vi "Read Data_HoldingRegistors.vi"(8 "error in (no error)":errorcluster, 11 "Device in":refnum<class "MB_TCP_Device.lvclass">) -> (0 "error out":errorcluster, 2 "AI Data":dbl[](array[numeric]), 3 "Device out":refnum<class "MB_TCP_Device.lvclass">)   [LabVIEW 2023, in "MB_TCP_Device.lvclass"]
uses:
  MB_TCP_Device.lvclass
  MB_TCP_Device.lvclass/MB_TCP_Device.ctl
  <vilib>/NI Modbus.llb/MB Ethernet Master Query Read Holding Registers (poly).vi
  <vilib>/Utility/error.llb/Error Cluster From Error Code.vi
  <vilib>/ErrorRing/Error Ring.xnode
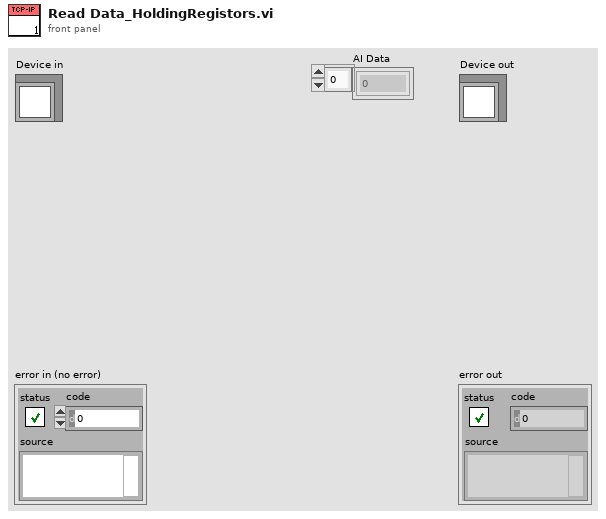
[diagram p1: front panel]
types:
  T1 = typedef "DAQ Device_IO ChannelsData.ctl" = cluster{"#DigitalInputs":u16, "StartAddress_DI":u16, "#DigitalOutputs":u16, "StartAddress_DO":u16, "#AnalogInputs":u16, "StartAddress_AI":u16, "#AnalogOutputs":u16, "StartAddress_AO":u16, "Coil_ReadData":bool[], "Coil_WriteData":bool[], "AI_Data":u16[], "AO_Data":u16[]}
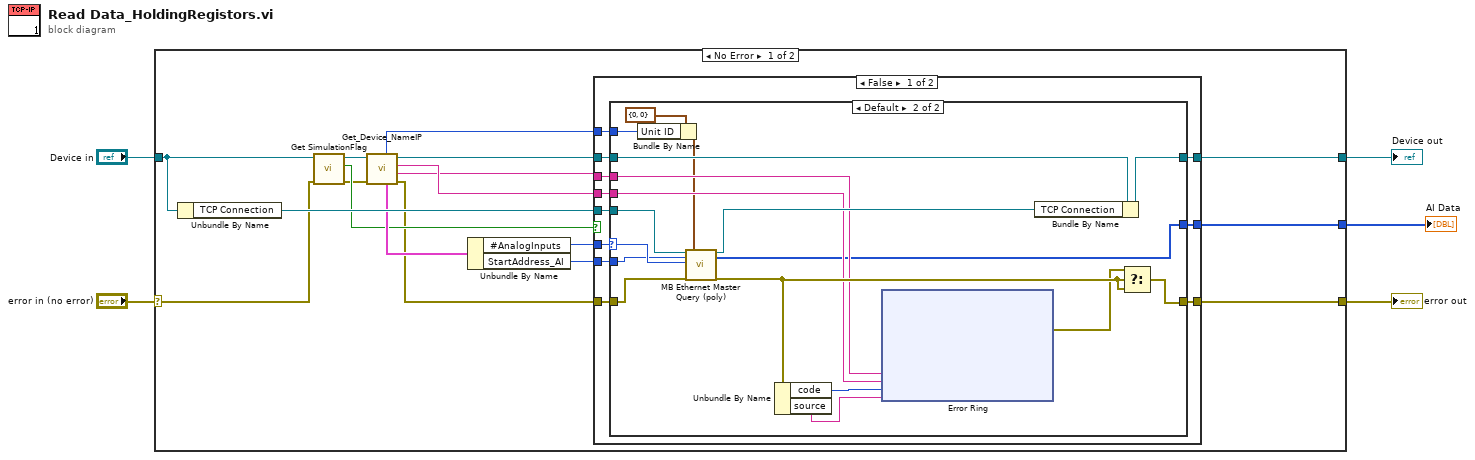
[diagram p0: block diagram]
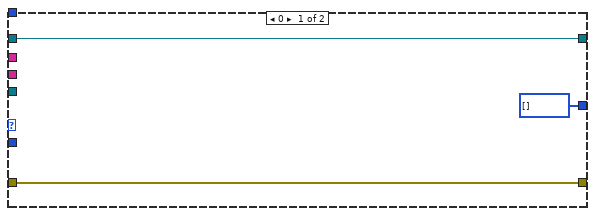
[diagram p2: hidden frame]
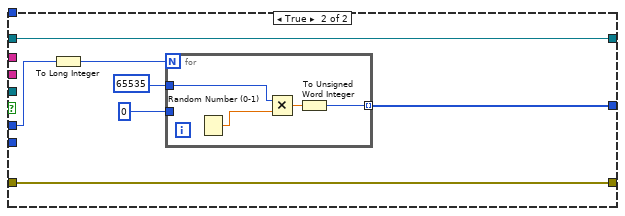
[diagram p3: hidden frame]
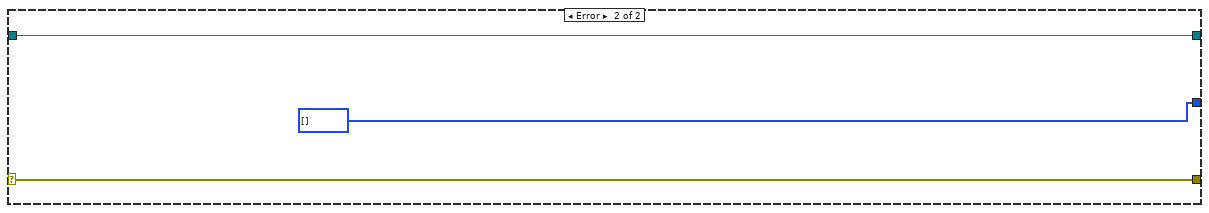
[diagram p4: hidden frame]
diagram:
  n1 = case shown="No Error" "error in (no error)" {
    selector: "error in (no error)" -> [w8 w78]
    tunnel: [w21 w78] -> w4
    tunnel: [w22 w77] -> w2
    tunnel: "Device in" -> [w14 w77]
    tunnel: [w6 u16[] [] ("register values")] -> w1
    frame No Error {
      n2 = Unbundle By Name(w14) -> ("TCP Connection"=w20:refnum<k5>)
      n3 = call-dynamic "Get SimulationFlag.vi"("error in (no error)"=w8, "Device in"=w14) -> ("error out"=w9:errorcluster, "Simulation?"=w12:bool, "Device out"=w15:refnum<class "MB_TCP_Device.lvclass">)  [unwired: 7 in]
      n4 = call-dynamic "Get_Device_NameIP.vi"("error in (no error)"=w9, "Device in"=w15) -> ("error out"=w7:errorcluster, "Device Name"=w17:string, "Device Address"=w18:string, "Device out"=w13:refnum<class "MB_TCP_Device.lvclass">, "IO Channels"=w19:T1, "Unit ID"=w16:u8)  [unwired: 4 in]
      n5 = Unbundle By Name(w19) -> ("#AnalogInputs"=w11:u16, "StartAddress_AI"=w10:u16)
      n6 = case shown="False" w12 {
        tunnel: [w33 w66] -> w22
        tunnel: w7 -> [w32 w71]
        tunnel: w11 -> [w25 w68]
        tunnel: w10 -> [w31 _]
        tunnel: [w30 w71] -> w21
        tunnel: w20 -> [w29 _]
        tunnel: w18 -> [w26 _]
        tunnel: w13 -> [w28 w66]
        tunnel: w17 -> [w27 _]
        tunnel: w16 -> [w24 _]
        tunnel: [w23 w65] -> w6
        frame False {
          n7 = case shown="Default" w25 {
            selector: w25 -> [_ w42]
            tunnel: [w36 w54] -> w33
            tunnel: w32 -> [w35 w52]
            tunnel: w31 -> [_ w41]
            tunnel: [w35 w50] -> w30
            tunnel: w29 -> [_ w49]
            tunnel: w28 -> [w36 w48]
            tunnel: w27 -> [_ w47]
            tunnel: w26 -> [_ w46]
            tunnel: w24 -> [_ w38]
            tunnel: [u16[] [] ("Holding Registers") w37] -> w23
            frame 0 {
            }
            frame Default {
              n8 = Bundle By Name(cluster=cluster{"Transaction ID":u16, "Unit ID":u8} {"Transaction ID"=0, "Unit ID"=0} ("MBAP Header"), "Unit ID"=w38) -> (w39:cluster{"Transaction ID":u16, "Unit ID":u8})
              n9 = call-poly <vilib>:"MB Ethernet Master Query (poly).vi"("TCP Connection Refnum in"=w49, "Starting Address"=w41, "Quantity"=w42, "error in"=w52, "MBAP Header"=w39) -> ("TCP Connection Refnum (dup)"=w53:refnum<k5>, "Holding Registers"=w37:u16[], "error out"=w51:errorcluster)  [unwired: 11 in, 1 out]
              n10 = Unbundle By Name(w51) -> ("code"=w45:i32, "source"=w44:string)
              n11 = xnode "Error Ring"("parameter 0"=w47, "parameter 1"=w46, "parameter 2"=w45, "parameter 3"=w44) -> ("error out"=w43:errorcluster)
              n12 = Bundle By Name(cluster=w48, "TCP Connection"=w53) -> (w54:refnum<class "MB_TCP_Device.lvclass">)
              n13 = Select(t=w43, s=w51, f=w51) -> (s? t:f=w50:errorcluster)
            }
          }
        }
        frame True {
          n14 = To Long Integer(number=w68) -> (32bit integer=w67:i32)
          n15 = for {
            N: w67 -> [_]
            tunnel: 65535 ("register") -> [w75]
            tunnel: 0 ("register") -> [_]
            tunnel: [w72] -> w65 mode=indexing
            n16 = Random Number (0-1)() -> (number: 0 to 1=w74:dbl)
            n17 = Multiply(x=w75, y=w74) -> (x*y=w73:dbl)
            n18 = To Unsigned Word Integer(number=w73) -> (unsigned 16bit integer=w72:u16)
          }
        }
      }
    }
    frame Error {
    }
  }
  "error out" <- w4
  "Device out" <- w2
  "AI Data" <- w1
